vi "add channel to configuration.vi"(8 "error in":errorcluster, 10 "TBM channel in":refnum<class "TBM channel.lvclass">, 11 "Tag Bus Web Interface configuration in":refnum<class "Tag Bus Web Interface configuration.lvclass">) -> (0 "error out":errorcluster, 3 "Tag Bus Web Interface configuration out":refnum<class "Tag Bus Web Interface configuration.lvclass">)   [LabVIEW 2013, in "Tag Bus Web Interface configuration.lvclass"]
uses:
  Tag Bus Web Interface configuration.lvclass
  <vilib>/NI/Tag Bus Module Framework/channel/TBM channel.lvclass
  <vilib>/NI/Tag Bus/tag/tag descriptor.lvclass/tag descriptor.ctl
  Tag Bus Web Interface configuration.lvclass/Tag Bus Web Interface configuration.ctl
  Read channels.vi
  Write channels.vi
  <vilib>/NI/Tag Bus/tag/read tag name.vi
  <vilib>/NI/Tag Bus/tag/tag descriptor.lvclass
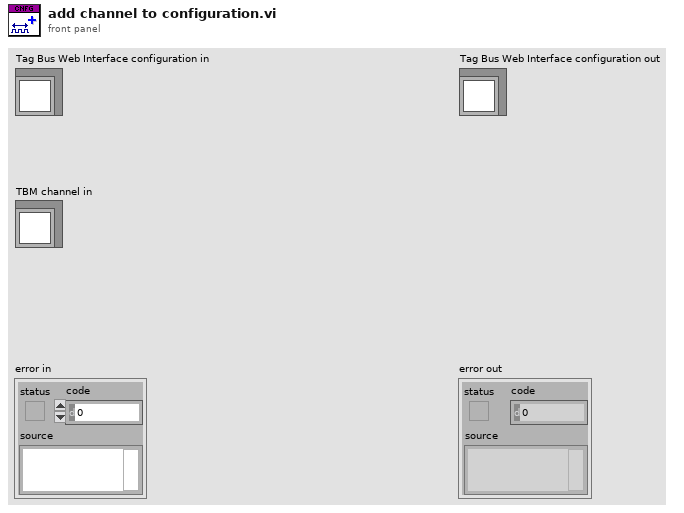
[diagram p1: front panel]
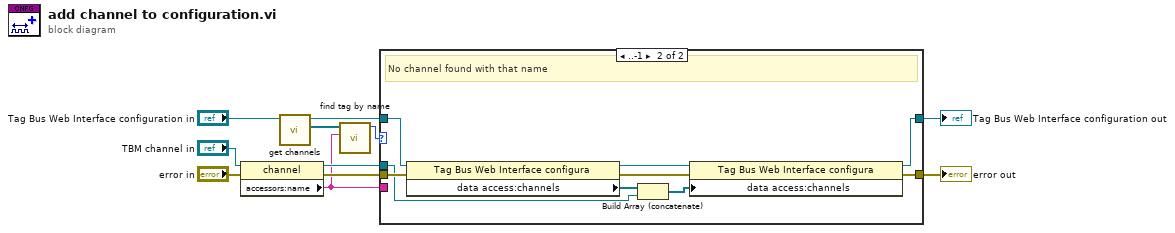
[diagram p0: block diagram]
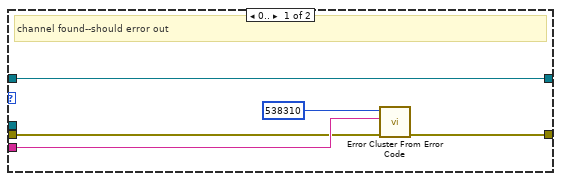
[diagram p2: hidden frame]
diagram:
  n1 = property class="channel"(reference="TBM channel in", error in="error in") -> (reference out=w10:refnum<class "TBM channel.lvclass">, error out=w7:errorcluster, "accessors:name"=w2:string)
  n2 = call-dynamic "get channels.vi"("Tag Bus Web Interface configuration in"="Tag Bus Web Interface configuration in") -> ("channels"=w3:refnum<class "TBM channel.lvclass">[], "Tag Bus Web Interface configuration out"=w11:refnum<class "Tag Bus Web Interface configuration.lvclass">)  [unwired: 9 in]
  n3 = call <vilib>:"find tag by name.vi"("name"=w2, "tags in"=w3) -> ("index"=w1:i32)  [unwired: 9 in]
  n4 = case shown="..-1" w1 {
    tunnel: [w16 w18] -> w6
    tunnel: w2 -> [w14 _]
    tunnel: w7 -> [w13 w25]
    tunnel: w11 -> [w12 w24]
    tunnel: w10 -> [_ w19]
    tunnel: [w12 w17] -> w5
    frame 0.. {
      # "channel found--should error out"
      n5 = call <vilib>:"Error Cluster From Error Code.vi"("error in (no error)"=w13, "error message (\"\")"=w14, "error code (0)"=538310) -> ("error out"=w16:errorcluster)  [unwired: 6 in]
    }
    frame ..-1 {
      # "No channel found with that name"
      n6 = property class="Tag Bus Web Interface configura"(reference=w24, error in=w25) -> (reference out=w23:refnum<class "Tag Bus Web Interface configuration.lvclass">, error out=w22:errorcluster, "data access:channels"=w21:refnum<class "TBM channel.lvclass">[])
      n7 = Build Array (concatenate)(w21, w19) -> (w20:refnum<class "TBM channel.lvclass">[])
      n8 = property class="Tag Bus Web Interface configura"(reference=w23, error in=w22, "data access:channels"=w20) -> (reference out=w17:refnum<class "Tag Bus Web Interface configuration.lvclass">, error out=w18:errorcluster)
    }
  }
  "error out" <- w6
  "Tag Bus Web Interface configuration out" <- w5
